vi "licz_fx.vi"(11 "Cluster":T1) -> (3 "f(x)":dbl)   [LabVIEW 2020]
doc: "liczenie wartość funkcji sześciennej od x"
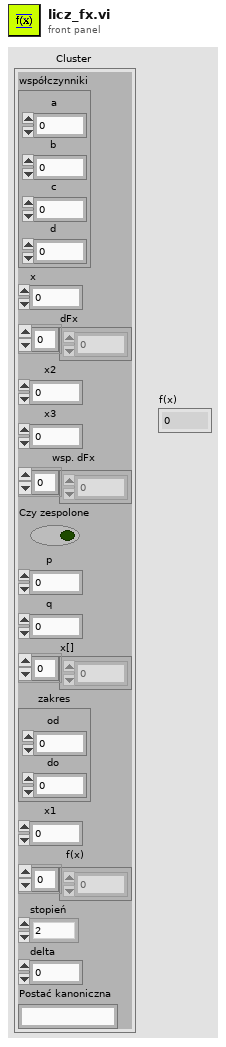
[diagram p1: front panel]
types:
  T1 = cluster{"współczynniki":cluster{"a":dbl, "b":dbl, "c":dbl, "d":dbl}, "x":dbl, "dFx":dbl[], "x2":cdb, "x3":cdb, "wsp. dFx":dbl[], "Czy zespolone":bool, "p":dbl, "q":dbl, "x[]":dbl[], "zakres":cluster{"od":dbl, "do":dbl}, "x1":cdb, "f(x)":dbl[], "stopień":enum16{"2", "3"}, "delta":i16, "Postać kanoniczna":string}
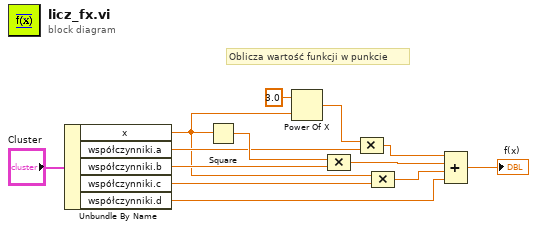
[diagram p0: block diagram]
diagram:
  # "Oblicza wartość funkcji w punkcie"
  n1 = Unbundle By Name("Cluster") -> ("x"=w4:dbl, "współczynniki.a"=w5:dbl, "współczynniki.b"=w11:dbl, "współczynniki.c"=w13:dbl, "współczynniki.d"=w7:dbl)
  n2 = Square(x=w4) -> (x^2=w10:dbl)
  n3 = Power Of X(1:w4, 2:3.0 ("y")) -> (0:w2:dbl)
  n4 = Compound Arithmetic op=MULTIPLY(w10, w11) -> (w9:dbl)
  n5 = Compound Arithmetic op=MULTIPLY(w2, w5) -> (w6:dbl)
  n6 = Compound Arithmetic op=MULTIPLY(w4, w13) -> (w12:dbl)
  n7 = Compound Arithmetic op=ADD(w6, w9, w12, w7) -> (→"f(x)":dbl)
